vi "CheckWhileMotion.vi"(6 "Motor":i32=1, 8 "error In":errorcluster, 9 "Device Address In":i32, 10 "DeviceKey In":string, 11 "CmdLib In":refnum<k24>) -> (0 "error Out":errorcluster, 1 "Device Address Out":i32, 2 "DeviceKey Out":string, 3 "CmdLib Out":refnum<k24>, 5 "Is Motion Done":bool)   [LabVIEW 2020]
uses:
  C:/GEECS/Developers Version/builds/Device builds/Picomotor8742dotNet/CmdLib.dll
  CmdLib.dll
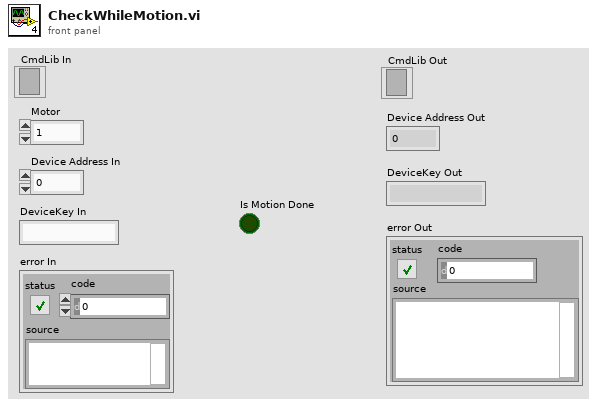
[diagram p1: front panel]
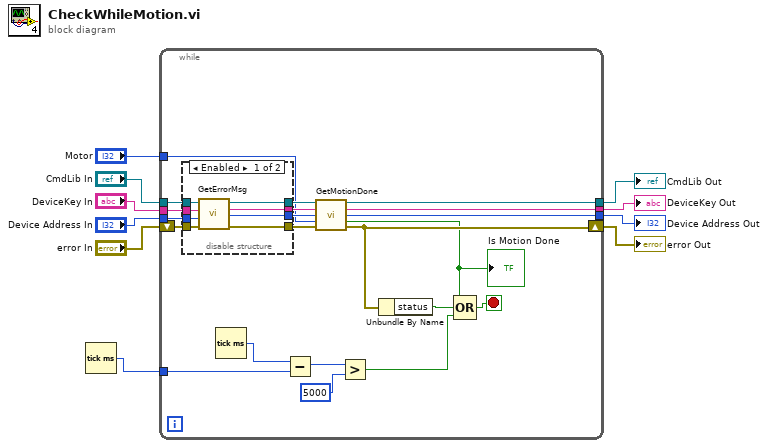
[diagram p0: block diagram]
diagram:
  n1 = Tick Count (ms)() -> (millisecond timer value=w1:u32)
  n2 = while {
    tunnel: "Motor" -> [w18]
    tunnel: "CmdLib In" -> [w29]
    tunnel: "DeviceKey In" -> [w28]
    tunnel: "Device Address In" -> [w25]
    shift-right: [w19] -> w3
    shift-left: "error In" -> [w27]
    tunnel: [w21] -> w5
    tunnel: [w22] -> w2
    tunnel: [w20] -> w4
    tunnel: w1 -> [w14]
    stop <- w23 stop-if-true
    n3 = disable-structure shown="Enabled" {
      disable-tunnel: [w39 w42] -> w31
      disable-tunnel: [w38 w43] -> w30
      disable-tunnel: w29 -> [w37 w43]
      disable-tunnel: w28 -> [w36 w42]
      disable-tunnel: w27 -> [w35 w40]
      disable-tunnel: [w34 w40] -> w26
      disable-tunnel: w25 -> [w33 w41]
      disable-tunnel: [w32 w41] -> w24
      frame Enabled {
        n4 = call "GetErrorMsg.vi"("error in (no error)"=w35, "Device Address In"=w33, "DeviceKey In"=w36, "CmdLib In"=w37) -> ("error out"=w34:errorcluster, "Device Address Out"=w32:i32, "DeviceKey Out"=w39:string, "CmdLib Out"=w38:refnum<k24>)
      }
      frame Disabled {
      }
    }
    n5 = Tick Count (ms)() -> (millisecond timer value=w15:u32)
    n6 = Subtract(x=w15, y=w14) -> (x-y=w13:u32)
    n7 = call "GetMotionDone.vi"("CmdLib In"=w30, "DeviceKey In"=w31, "Device Address In"=w24, "Motor"=w18, "error in (no error)"=w26) -> ("CmdLib Out"=w22:refnum<k24>, "DeviceKey Out"=w21:string, "Device Address Out"=w20:i32, "Is Motion Done"=w17:bool, "error out"=w19:errorcluster)  [unwired: 6 in]
    "Is Motion Done" <- w17
    n8 = Greater?(x=w13, y=u32 5000) -> (0:w11:bool)
    n9 = Unbundle By Name(w19) -> ("status"=w16:bool)
    n10 = Compound Arithmetic op=OR(w17, w16, w11) -> (w23:bool)
  }
  "CmdLib Out" <- w2
  "DeviceKey Out" <- w5
  "Device Address Out" <- w4
  "error Out" <- w3
